vi "Get Neuron Properties.vi"(11 "Neuron in":refnum<class "Neuron.lvclass">) -> (0 "Position Key":i32, 1 "Active":bool, 2 "InGROUP ID":i32, 3 "Neuron out":refnum<class "Neuron.lvclass">, 4 "Group":T1, 5 "ID":i32)   [LabVIEW 2013, in "Neuron.lvclass"]
doc: "Read the properties of a Neuron"
uses:
  Neuron.lvclass
  Controls/Type of Neuron.ctl
  Neuron.lvclass/Neuron.ctl
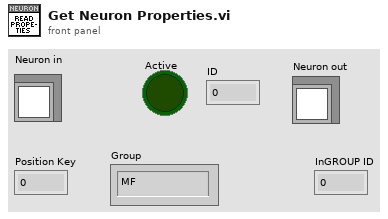
[diagram p1: front panel]
types:
  T1 = typedef "Type of Neuron.ctl" = enum16{"MF", "BA", "GO", "GC", "PC", "LU", "Glia (Dummy)"}
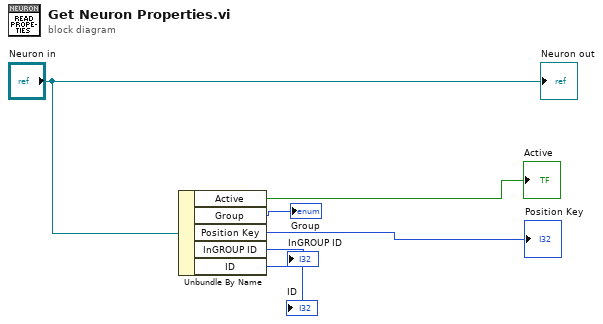
[diagram p0: block diagram]
diagram:
  n1 = Unbundle By Name("Neuron in") -> ("Active"=→"Active":bool, "Group"=→"Group":T1, "Position Key"=→"Position Key":i32, "InGROUP ID"=→"InGROUP ID":i32, "ID"=→"ID":i32)
  "Neuron out" <- "Neuron in"
